vi "Cleanup.vi"(8 "error in (no error)":errorcluster, 11 "Team Config Panel in":refnum<class "Team Config Panel.lvclass">) -> (0 "error out":errorcluster)   [LabVIEW 2020, in "SB App.lvlib" / "Team Config Panel.lvclass"]
uses:
  Team Config Panel.lvclass
  Team Config Panel.lvclass/Team Config Panel.ctl
  <vilib>/IlluminatedG/IG OOPanel/OOPanel/ArrayPanel/ArrayPanel.lvclass
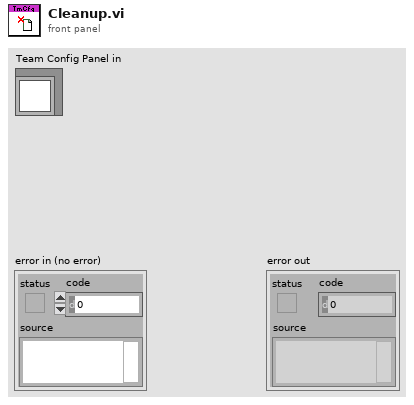
[diagram p1: front panel]
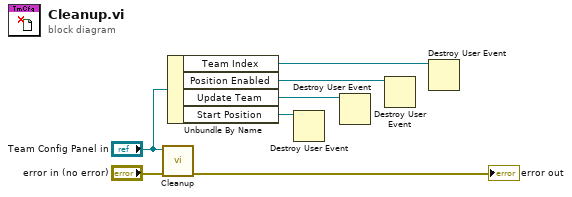
[diagram p0: block diagram]
diagram:
  n1 = call-parent "Cleanup.vi"("error in (no error)"="error in (no error)", "ArrayPanel in"="Team Config Panel in") -> ("error out"=→"error out":errorcluster)  [unwired: 9 in]
  n2 = Unbundle By Name("Team Config Panel in") -> ("Team Index"=w1:refnum<user-event>, "Position Enabled"=w2:refnum<user-event>, "Update Team"=w3:refnum<user-event>, "Start Position"=w4:refnum<user-event>)
  n3 = Destroy User Event(user event=w4) -> ()  [unwired: 1 in, 1 out]
  n4 = Destroy User Event(user event=w3) -> ()  [unwired: 1 in, 1 out]
  n5 = Destroy User Event(user event=w2) -> ()  [unwired: 1 in, 1 out]
  n6 = Destroy User Event(user event=w1) -> ()  [unwired: 1 in, 1 out]
